vi "go to hold from ll.vi"(0 "system status in":T2={"system state"=enum."Empty & Closed", "fuel level"=0.0, "LOX level"=0.0, "system warnings"={"oxidizer overpress"=FALSE, "oxidizer leak"=FALSE, "fuel overpress"=FALSE, "fuel leak"=FALSE}, "valves"={"fuel load"=FALSE, "fuel return"=FALSE, "fuel comb"=FALSE, "fuel dump"=FALSE, "LOX load"=FALSE, "LOX return"=FALSE, "LOX comb"=FALSE, "LOX dump"=FALSE}, "ignition"=FALSE}, 11 "rocket controls":T1, 13 "LOX leak":bool, 15 "fuel leak":bool) -> (4 "system status out":T2={"system state"=enum."Empty & Closed", "fuel level"=0.0, "LOX level"=0.0, "system warnings"={"oxidizer overpress"=FALSE, "oxidizer leak"=FALSE, "fuel overpress"=FALSE, "fuel leak"=FALSE}, "valves"={"fuel load"=FALSE, "fuel return"=FALSE, "fuel comb"=FALSE, "fuel dump"=FALSE, "LOX load"=FALSE, "LOX return"=FALSE, "LOX comb"=FALSE, "LOX dump"=FALSE}, "ignition"=FALSE})   [LabVIEW 2017]
doc: "This subVI handles the logic going to the hold state from the load fuel state for the rocket engine simulation.\nIt sets the state enum to the hold state when the fuel level is 100, or if hold is pushed, or if a leak is detected in either tank.\n\nPaul K Dixon\nP350\nCSUSB"
uses:
  typedefs/sysyem status.ctl
  typedefs/system state.ctl
  typedefs/rocket system warnings.ctl
  typedefs/user controls.ctl
panel:
  # "Standard\nProcedures"
  # "Alternate\nProcedures"
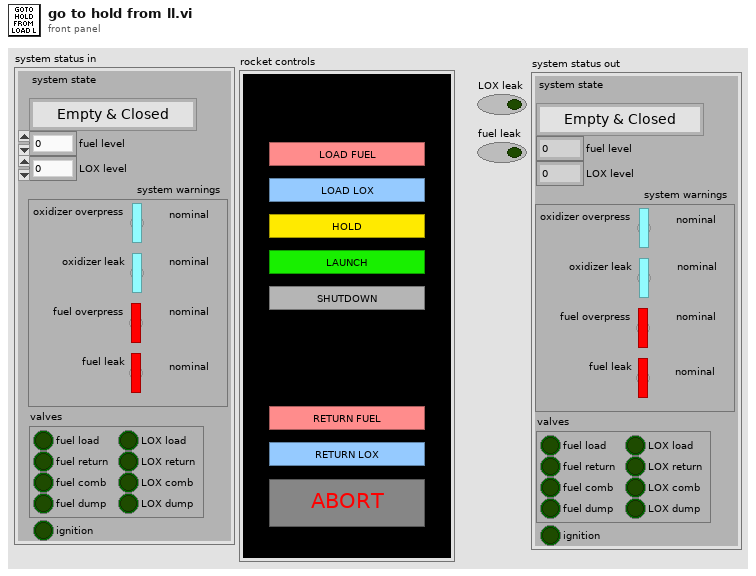
[diagram p1: front panel]
types:
  T1 = typedef "user controls.ctl" = cluster{"load fuel":bool, "load lox":bool, "hold":bool, "launch":bool, "shutdown":bool, "return fuel":bool, "return lox":bool, "abort":bool}
  T2 = typedef "sysyem status.ctl" = cluster{"system state":T3, "fuel level":dbl, "LOX level":dbl, "system warnings":T4, "valves":cluster{"fuel load":bool, "fuel return":bool, "fuel comb":bool, "fuel dump":bool, "LOX load":bool, "LOX return":bool, "LOX comb":bool, "LOX dump":bool}, "ignition":bool}
  T3 = typedef "system state.ctl" = enum16{"Hold", "Empty & Closed", "Launch", "Return Fuel", "Return LOX", "Loading Lox", "Loading Fuel", "Shutdown", "Abort"}
  T4 = typedef "rocket system warnings.ctl" = cluster{"oxidizer overpress":bool, "oxidizer leak":bool, "fuel overpress":bool, "fuel leak":bool}
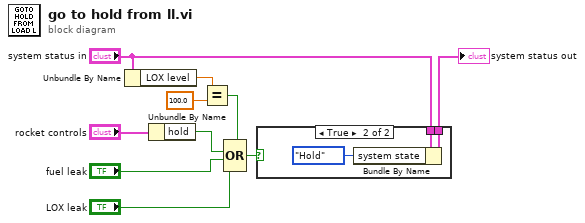
[diagram p0: block diagram]
diagram:
  n1 = Unbundle By Name("system status in") -> ("LOX level"=w3:dbl)
  n2 = Unbundle By Name("rocket controls") -> ("hold"=w7:bool)
  n3 = Equal?(x=w3, y=100.0) -> (x = y?=w2:bool)
  n4 = Compound Arithmetic op=OR(w2, w7, "fuel leak", "LOX leak") -> (w9:bool)
  n5 = case shown="True" w9 {
    tunnel: "system status in" -> [w11 w14]
    tunnel: [w11 w13] -> w10
    frame False {
    }
    frame True {
      n6 = Bundle By Name(cluster=w14, "system state"=system_state."Hold") -> (w13:T2)
    }
  }
  "system status out" <- w10
